vi "GetValue.vi"(8 "error in":errorcluster, 11 "Measure in":refnum<class "MeasureKind.lvclass">) -> (0 "error out":errorcluster, 2 "Value":T1, 3 "Measure out":refnum<class "MeasureKind.lvclass">)   [LabVIEW 2021, in "ProligentXMLGenerator.lvlib" / "MeasureKind.lvclass"]
uses:
  MeasureKind.lvclass
  MeasureKind.lvclass/MeasureKind.ctl
  Value.ctl
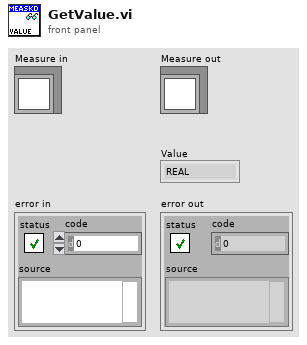
[diagram p1: front panel]
types:
  T1 = typedef "ProligentXMLGenerator.lvlib/MeasureKind.lvclass/Value.ctl" = enum16{"REAL", "BOOL", "INTEGER", "STRING", "DATETIME"}
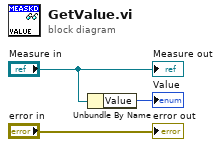
[diagram p0: block diagram]
diagram:
  n1 = Unbundle By Name("Measure in") -> ("Value"=→"Value":T1)
  "error out" <- "error in"
  "Measure out" <- "Measure in"
